vi "run_BuildAll.vi"(8 "error in (no error)":errorcluster, 10 "name or relative path":string, 11 "Workspace path":path) -> (0 "error out":errorcluster)   [LabVIEW 2016]
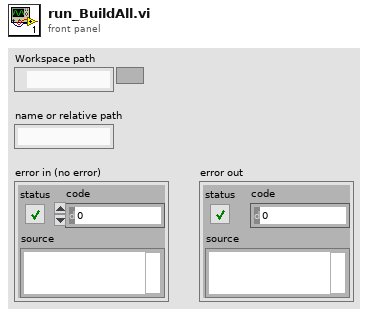
[diagram p1: front panel]
types:
  T1 = enum32{"Invalid", "Standard", "Closed", "Hidden", "Minimized", "Maximized"}
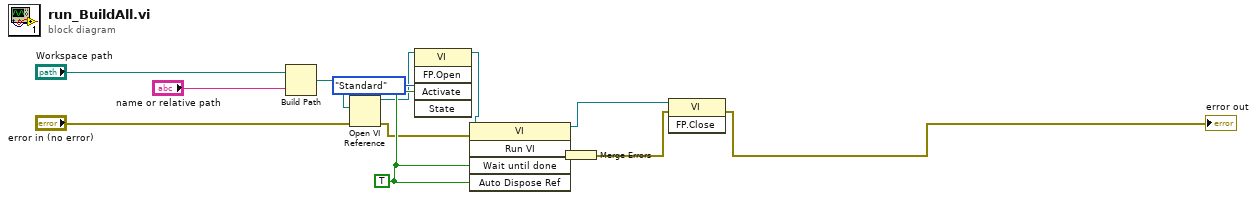
[diagram p0: block diagram]
diagram:
  w9 = TRUE ("Wait Until Done")
  n1 = Build Path(base path="Workspace path", name or relative path="name or relative path") -> (appended path=w3:path)
  n2 = Open VI Reference(vi path=w3, error in (no error)="error in (no error)") -> (vi reference=w7:refnum<vi>, error out=w5:errorcluster)  [unwired: 4 in]
  n3 = invoke class="VI" method="FP.Open"(reference=w7, "Activate"=w9, "State"=T1."Standard") -> (reference out=w8:refnum<vi>)  [unwired: 2 in, 4 out]
  n4 = invoke class="VI" method="Run VI"(reference=w8, error in=w5, "Wait until done"=w9, "Auto Dispose Ref"=w9) -> (reference out=w11:refnum<vi>, error out=w6:errorcluster)  [unwired: 1 in, 3 out]
  n5 = Merge Errors(w6) -> (w12:errorcluster)
  n6 = invoke class="VI" method="FP.Close"(reference=w11, error in=w12) -> (error out=→"error out":errorcluster)  [unwired: 1 in, 2 out]
